vi "ReadL.vi"(8 "error in (no error)":errorcluster, 10 "Offset":u32) -> (0 "error out":errorcluster, 2 "Data 2":u32=255, 3 "Data 1":u32=255)   [LabVIEW 2015, in "ESLSCDLL.lvlib"]
uses:
  ESLSCDLL.lvlib
  Globals.vi
  ESLSCDLL.dll
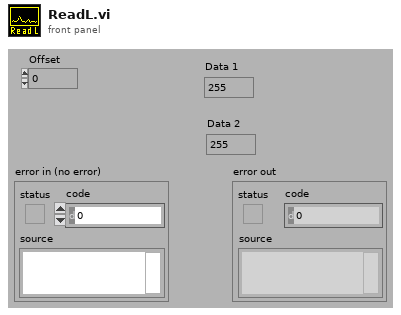
[diagram p1: front panel]
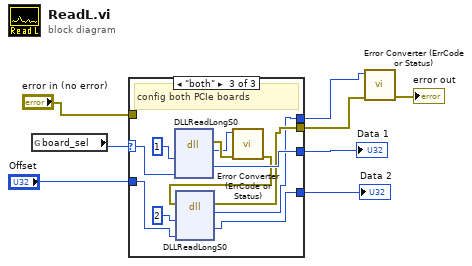
[diagram p0: block diagram]
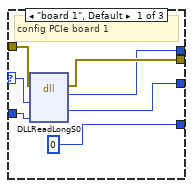
[diagram p2: hidden frame]
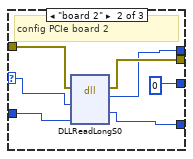
[diagram p3: hidden frame]
diagram:
  n1 = global read "Globals.vi" "board_sel"() -> (w1:enum32{"0", "board 1", "board 2", "both"})
  n2 = case shown="\"both\"" w1 {
    selector: w1 -> [w13 w21 w28]
    tunnel: [w15 u32 0 w33] -> w8
    tunnel: "Offset" -> [w14 w20 w31]
    tunnel: [u32 0 w22 w32] -> w7
    tunnel: "error in (no error)" -> [w11 w18 _]
    tunnel: [w10 w17 w24] -> w3
    tunnel: [w9 w16 w23] -> w2
    frame "board 1", Default {
      # "config PCIe board 1"
      n3 = dll-call lib="C:/ENTW/PCIE/LV64/board.vis/ESLSCDLL.dll" fn="DLLReadLongS0"(error in=w11, "drv"=w13, "PortOff"=w14) -> (error out=w10:errorcluster, "es_status_codes"=w9:i32, "data"=w15:u32)  [unwired: 5 in, 1 out]
    }
    frame "board 2" {
      # "config PCIe board 2"
      n4 = dll-call lib="C:/ENTW/PCIE/LV64/board.vis/ESLSCDLL.dll" fn="DLLReadLongS0"(error in=w18, "drv"=w21, "PortOff"=w20) -> (error out=w17:errorcluster, "es_status_codes"=w16:i32, "data"=w22:u32)  [unwired: 5 in, 1 out]
    }
    frame "both" {
      # "config both PCIe boards"
      n5 = dll-call lib="C:/ENTW/PCIE/LV64/board.vis/ESLSCDLL.dll" fn="DLLReadLongS0"("drv"=u32 1, "PortOff"=w28) -> (error out=w27:errorcluster, "es_status_codes"=w26:i32, "data"=w33:u32)  [unwired: 6 in, 1 out]
      n6 = call "Error Converter (ErrCode or Status).vi"("error in (no error)"=w27, "error code"=w26) -> ("error out"=w25:errorcluster)  [unwired: 9 in]
      n7 = dll-call lib="C:/ENTW/PCIE/LV64/board.vis/ESLSCDLL.dll" fn="DLLReadLongS0"(error in=w25, "drv"=u32 2, "PortOff"=w31) -> (error out=w24:errorcluster, "es_status_codes"=w23:i32, "data"=w32:u32)  [unwired: 5 in, 1 out]
    }
  }
  "Data 1" <- w8
  "Data 2" <- w7
  n8 = call "Error Converter (ErrCode or Status).vi"("error in (no error)"=w3, "error code"=w2) -> ("error out"=→"error out":errorcluster)  [unwired: 9 in]
